vi "CTR_Network-Stream_Reader-Writer.vi"(8 "DAQ Endpoint":string, 9 "CTR Endpoint":string="CTR001", 10 "DAQ IP Addr":string, 11 "CTR IP Addr":string) -> (0 "//CTR IP Addr:CTR000/DAQ000-Data":string, 1 "//DAQ IP Addr:DAQ000/DAQ000-Data":string, 2 "//CTR IP Addr:CTR000/DAQ000-Control":string, 3 "//DAQ IP Addr:DAQ000/DAQ000-Control":string)   [LabVIEW 2024]
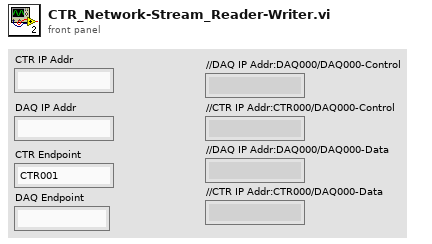
[diagram p1: front panel]
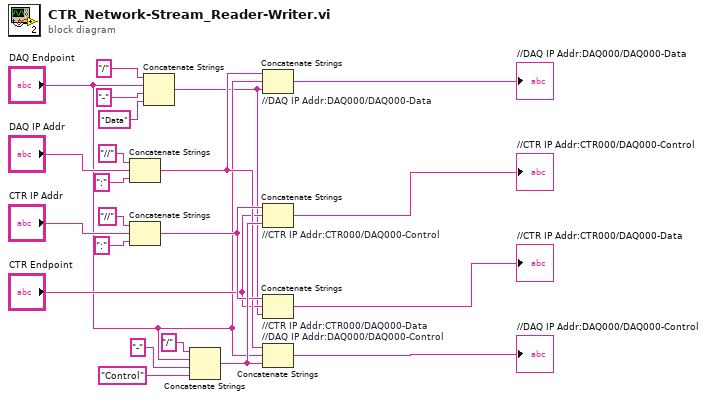
[diagram p0: block diagram]
diagram:
  n1 = Concatenate Strings("//" ("string"), "DAQ IP Addr", ":" ("string")) -> (w6:string)
  n2 = Concatenate Strings("//" ("string"), "CTR IP Addr", ":" ("string")) -> (w7:string)
  n3 = Concatenate Strings("/" ("string"), "DAQ Endpoint", "-" ("string"), "Data" ("string")) -> (w3:string)
  n4 = Concatenate Strings("/" ("string"), "DAQ Endpoint", "-" ("string"), "Control" ("string")) -> (w18:string)
  n5 = Concatenate Strings "//DAQ IP Addr:DAQ000/DAQ000-Data"(w6, "DAQ Endpoint", w3) -> (→"//DAQ IP Addr:DAQ000/DAQ000-Data":string)
  n6 = Concatenate Strings "//CTR IP Addr:CTR000/DAQ000-Control"(w7, "CTR Endpoint", w18) -> (→"//CTR IP Addr:CTR000/DAQ000-Control":string)
  n7 = Concatenate Strings "//CTR IP Addr:CTR000/DAQ000-Data"(w7, "CTR Endpoint", w3) -> (→"//CTR IP Addr:CTR000/DAQ000-Data":string)
  n8 = Concatenate Strings "//DAQ IP Addr:DAQ000/DAQ000-Control"(w6, "DAQ Endpoint", w18) -> (→"//DAQ IP Addr:DAQ000/DAQ000-Control":string)
